vi "Initialize Attributes.vi"(8 "error in (no error)":errorcluster, 10 "Attribute Data":variant, 11 "IVI_Counter in":refnum<class "IVI_Counter.lvclass">) -> (0 "error out":errorcluster, 2 "Found?":bool, 3 "IVI_Counter out":refnum<class "IVI_Counter.lvclass">)   [LabVIEW 2013, in "IVI_Counter.lvlib" / "IVI_Counter.lvclass"]
doc: "Initialize object attribute.\n\nUnique resources should be allocated elsewhere!"
uses:
  IVI_Counter.lvclass
  CSPP_Core/Actors/CS++DeviceActor/CS++DeviceActor.lvclass
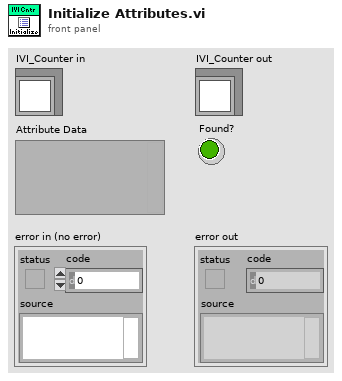
[diagram p1: front panel]
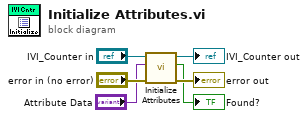
[diagram p0: block diagram]
diagram:
  n1 = call-parent "Initialize Attributes.vi"("error in (no error)"="error in (no error)", "Attribute Data"="Attribute Data", "CS++DeviceActor in"="IVI_Counter in") -> ("error out"=→"error out":errorcluster, "Found?"=→"Found?":bool, "CS++DeviceActor out"=→"IVI_Counter out":refnum<class "IVI_Counter.lvclass">)  [unwired: 6 in]
